vi "Glimpse get users directory names.vi"(0 "RAID root path":path, 1 "error in":errorcluster) -> (2 "Username":string, 3 "directory names":string[](array[string]), 4 "error out":errorcluster)   [LabVIEW 2016]
doc: "Returns the names of the acquisition directories in RAID root path that are prefaced by the username. If RAID root path is null returns no names."
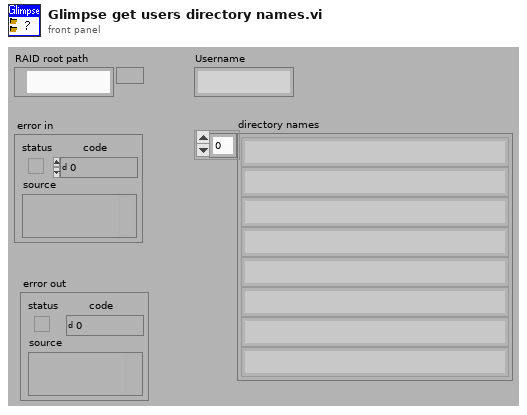
[diagram p1: front panel]
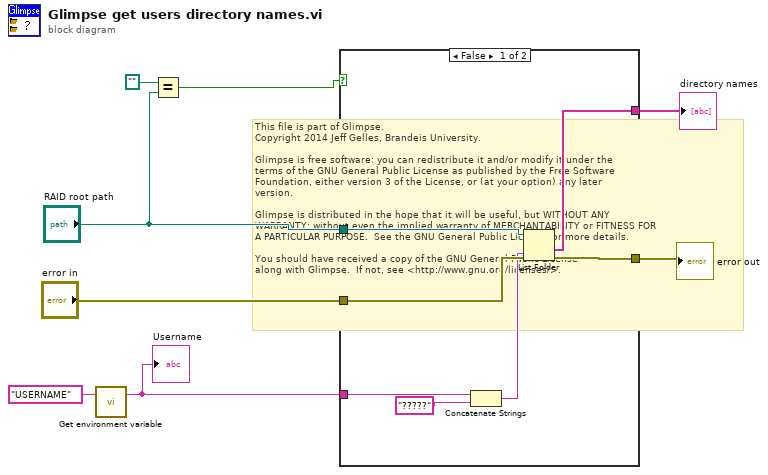
[diagram p0: block diagram]
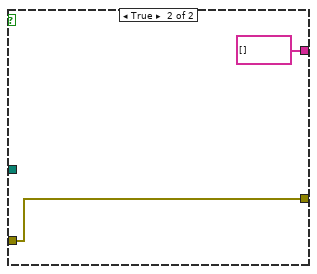
[diagram p2: hidden frame]
diagram:
  # "This file is part of Glimpse. \nCopyright 2014 Jeff Gelles, Brandeis University.    \n\nGlimpse is free software: you can redistribute it and/or modify it under the \nterms of the GNU General Public License as published by the Free Software \nFoundation, either version 3 of the License, or (at your option) any later \nversion.\n\nGlimpse is distributed in the hope that it will be useful, but WITHOUT ANY \nWARRANTY; without even the implied warranty of MERCHANTABILITY or FITNESS FOR \nA PARTICULAR PURPOSE.  See the GNU General Public License for more details.\n\nYou should have received a copy of the GNU General Public License\nalong with Glimpse.  If not, see <http://www.gnu.org/licenses/>."
  n1 = call "Get environment variable.vi"("Variable name"="USERNAME") -> ("Value"=w6:string)  [unwired: 2 out]
  "Username" <- w6
  n2 = Equal?(x=path "", y="RAID root path") -> (x = y?=w1:bool)
  n3 = case shown="False" w1 {
    tunnel: [w15 string[] [] ("folder names")] -> w8
    tunnel: [w14 w16] -> w7
    tunnel: w6 -> [w13 _]
    tunnel: "error in" -> [w12 w16]
    tunnel: "RAID root path" -> [w9 _]
    frame False {
      n4 = Concatenate Strings(w13, "?????" ("string")) -> (w11:string)
      n5 = List Folder(path=w9, pattern=w11, error in=w12) -> (folder names=w15:string[], error out=w14:errorcluster)  [unwired: 3 out]
    }
    frame True {
    }
  }
  "directory names" <- w8
  "error out" <- w7
